vi "Utility - Delete Empty Rows or Columns.vi"(2 "Delete Option":T1(ring), 3 "Array In":string[][](array[string])) -> (1 "Array Out":string[][](array[string]))   [LabVIEW 2019]
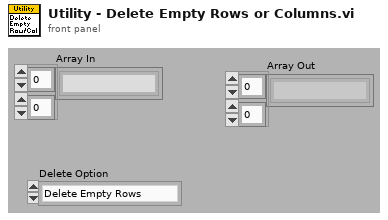
[diagram p1: front panel]
types:
  T1 = enum16{"Delete Empty Rows", "Delete Empty Columns"}
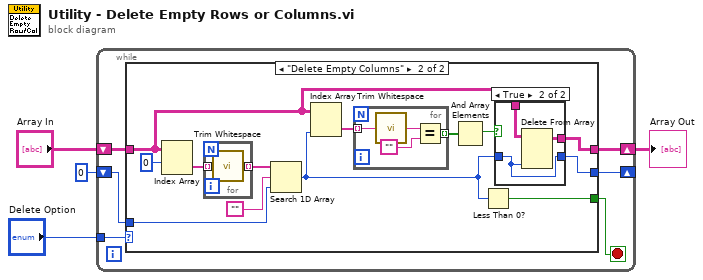
[diagram p0: block diagram]
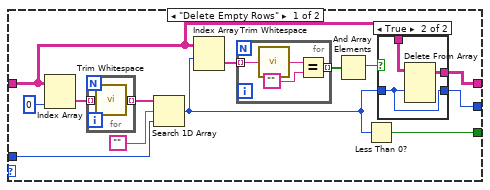
[diagram p2: hidden frame]
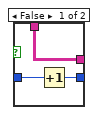
[diagram p3: hidden frame]
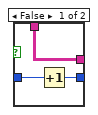
[diagram p4: hidden frame]
diagram:
  n1 = while {
    shift-right: [w9] -> w4
    shift-left: "Array In" -> [w10]
    tunnel: "Delete Option" -> [w8]
    shift-right: [w7] -> _
    shift-left: 0 ("index of element") -> [w6]
    stop <- w5 stop-if-true
    n2 = case shown="\"Delete Empty Columns\"" w8 {
      tunnel: w10 -> [w14 w41]
      tunnel: [w22 w47] -> w9
      tunnel: [w21 w46] -> w5
      tunnel: [w12 w39] -> w7
      tunnel: w6 -> [w11 w38]
      frame "Delete Empty Rows" {
        n3 = Index Array(array=w14, index (col)=0 ("index (row)")) -> (element=w18:string[])  [unwired: 1 in]
        n4 = for {
          tunnel: w18 -> [w35] mode=indexing
          tunnel: [w34] -> w19 mode=indexing
          n5 = call <vilib>:"Trim Whitespace.vi"("string"=w35) -> ("trimmed string"=w34:string)  [unwired: 1 in]
        }
        n6 = Search 1D Array(1D array=w19, element="", start index (0)=w11) -> (index of element=w16:i32)
        n7 = Index Array(array=w14, index (row)=w16) -> (element=w17:string[])  [unwired: 1 in]
        n8 = for {
          tunnel: w17 -> [w33] mode=indexing
          tunnel: [w30] -> w15 mode=indexing
          n9 = call <vilib>:"Trim Whitespace.vi"("string"=w33) -> ("trimmed string"=w32:string)  [unwired: 1 in]
          n10 = Equal?(x=w32, y="") -> (x = y?=w30:bool)
        }
        n11 = And Array Elements(Boolean array=w15) -> (logical AND=w13:bool)
        n12 = Less Than 0?(x=w16) -> (x < 0?=w21:bool)
        n13 = case shown="True" w13 {
          tunnel: [w26 w29] -> w22
          tunnel: w16 -> [w25 w27]
          tunnel: w14 -> [w26 w28]
          tunnel: [w24 w27] -> w12
          frame False {
            n14 = Increment(x=w25) -> (x+1=w24:i32)
          }
          frame True {
            n15 = Delete From Array(array=w28, index (row)=w27) -> (array with subset deleted=w29:string[][])  [unwired: 2 in, 1 out]
          }
        }
      }
      frame "Delete Empty Columns" {
        n16 = Index Array(array=w41, index (row)=0) -> (element=w44:string[])  [unwired: 1 in]
        n17 = for {
          tunnel: w44 -> [w60] mode=indexing
          tunnel: [w59] -> w45 mode=indexing
          n18 = call <vilib>:"Trim Whitespace.vi"("string"=w60) -> ("trimmed string"=w59:string)  [unwired: 1 in]
        }
        n19 = Search 1D Array(1D array=w45, element="", start index (0)=w38) -> (index of element=w37:i32)
        n20 = Index Array(array=w41, index (col)=w37) -> (element=w43:string[])  [unwired: 1 in]
        n21 = for {
          tunnel: w43 -> [w58] mode=indexing
          tunnel: [w55] -> w42 mode=indexing
          n22 = call <vilib>:"Trim Whitespace.vi"("string"=w58) -> ("trimmed string"=w57:string)  [unwired: 1 in]
          n23 = Equal?(x=w57, y="") -> (x = y?=w55:bool)
        }
        n24 = And Array Elements(Boolean array=w42) -> (logical AND=w40:bool)
        n25 = Less Than 0?(x=w37) -> (x < 0?=w46:bool)
        n26 = case shown="True" w40 {
          tunnel: [w51 w54] -> w47
          tunnel: w37 -> [w50 w52]
          tunnel: w41 -> [w51 w53]
          tunnel: [w49 w52] -> w39
          frame False {
            n27 = Increment(x=w50) -> (x+1=w49:i32)
          }
          frame True {
            n28 = Delete From Array(array=w53, index (col)=w52) -> (array with subset deleted=w54:string[][])  [unwired: 2 in, 1 out]
          }
        }
      }
    }
  }
  "Array Out" <- w4
